vi "Auto_Path Tracking_edit.vi"() -> ()   [LabVIEW 2020]
uses:
  <vilib>/Utility/file.llb/Read Delimited Spreadsheet (DBL).vi
  <vilib>/Instr/_visa.llb/VISA Configure Serial Port (Instr).vi
panel:
  in  "Tab Control":enum32{"GPS", "LiDAR (TRUE)", "ETC"}(tab)
  out "XYGraph":cluster{"array":dbl[], "array":dbl[]}[](graph)
  in  "COM":refnum<visa-resource-name>
  out "도분초(lon)":string
  out "도(lon)":string
  out "도분초(lat)":string
  out "도(lat)":string
  out "Latitude":dbl
  out "Longtitude":dbl
  out "UTC":dbl
  out "TM_X":dbl format="%#_6f"
  out "TM_Y":dbl format="%#_6f"
  in  "Refresh 2":bool
  out "WP_no. 2":i32
  out "Satellited Used":string
  out "Fix Position":string
  out "True_Heading":dbl
  out "velocity":dbl
  out "read buffer":string
  out "Safe Box Plotting":cluster{dbl[], dbl[]}[](graph)
  out "Clustering graph":T1(graph)
  out "XY graph":cluster{"X":dbl, "Y":dbl}[](graph)
  out "Box Point Array":cluster{dbl[], dbl[]}[](array[cluster])
  out "XY DATA":cluster{"X":dbl, "Y":dbl}[](array[cluster])
  out "Path_Vel_arr 2":dbl[](array[numeric])
  out "Path_long_arr 2":dbl[](array[numeric])
  out "Path_lat_arr 2":dbl[](array[numeric])
  out "x_lat_path 2":dbl[](array[numeric])
  out "y_long_path 2":dbl[](array[numeric])
  out "vel. path 2":dbl[](array[numeric])
  in  "?":enum32{"State", "ETC"}(tab)
  in  "stop":bool
  in  "file path (dialog if empty)":path=path "C:/Users/Mondicht Shin/Desktop/ERP42_Auto_TEST/RDDF_3_수정.txt" caption="RDDF"
  out "XY Graph":T2(graph)
  in  "Refresh":bool
  in  "A/M":bool=TRUE
  in  "Serial Name":refnum<visa-resource-name>="COM8"
  out "ERP_Serial_DATA(RAW)":string
  in  "Vel":dbl=4.0 format="%#_13g"
  out "Index(near vehicle)":i32
  out "WP_no.":i32
  out "Tracking_Error(m)":dbl
  out "x_lat_path":dbl[](array[numeric])
  out "y_long_path":dbl[](array[numeric])
  out "vel. path":dbl[](array[numeric])
  out "Path_Vel_arr":dbl[](array[numeric])
  out "Path_long_arr":dbl[](array[numeric])
  out "Path_lat_arr":dbl[](array[numeric])
  out "ERP_Receive":T3
  out "Steer_CMD(Deg)":dbl
  out "CMD_2_ERP":T4
  out "Brake":u8
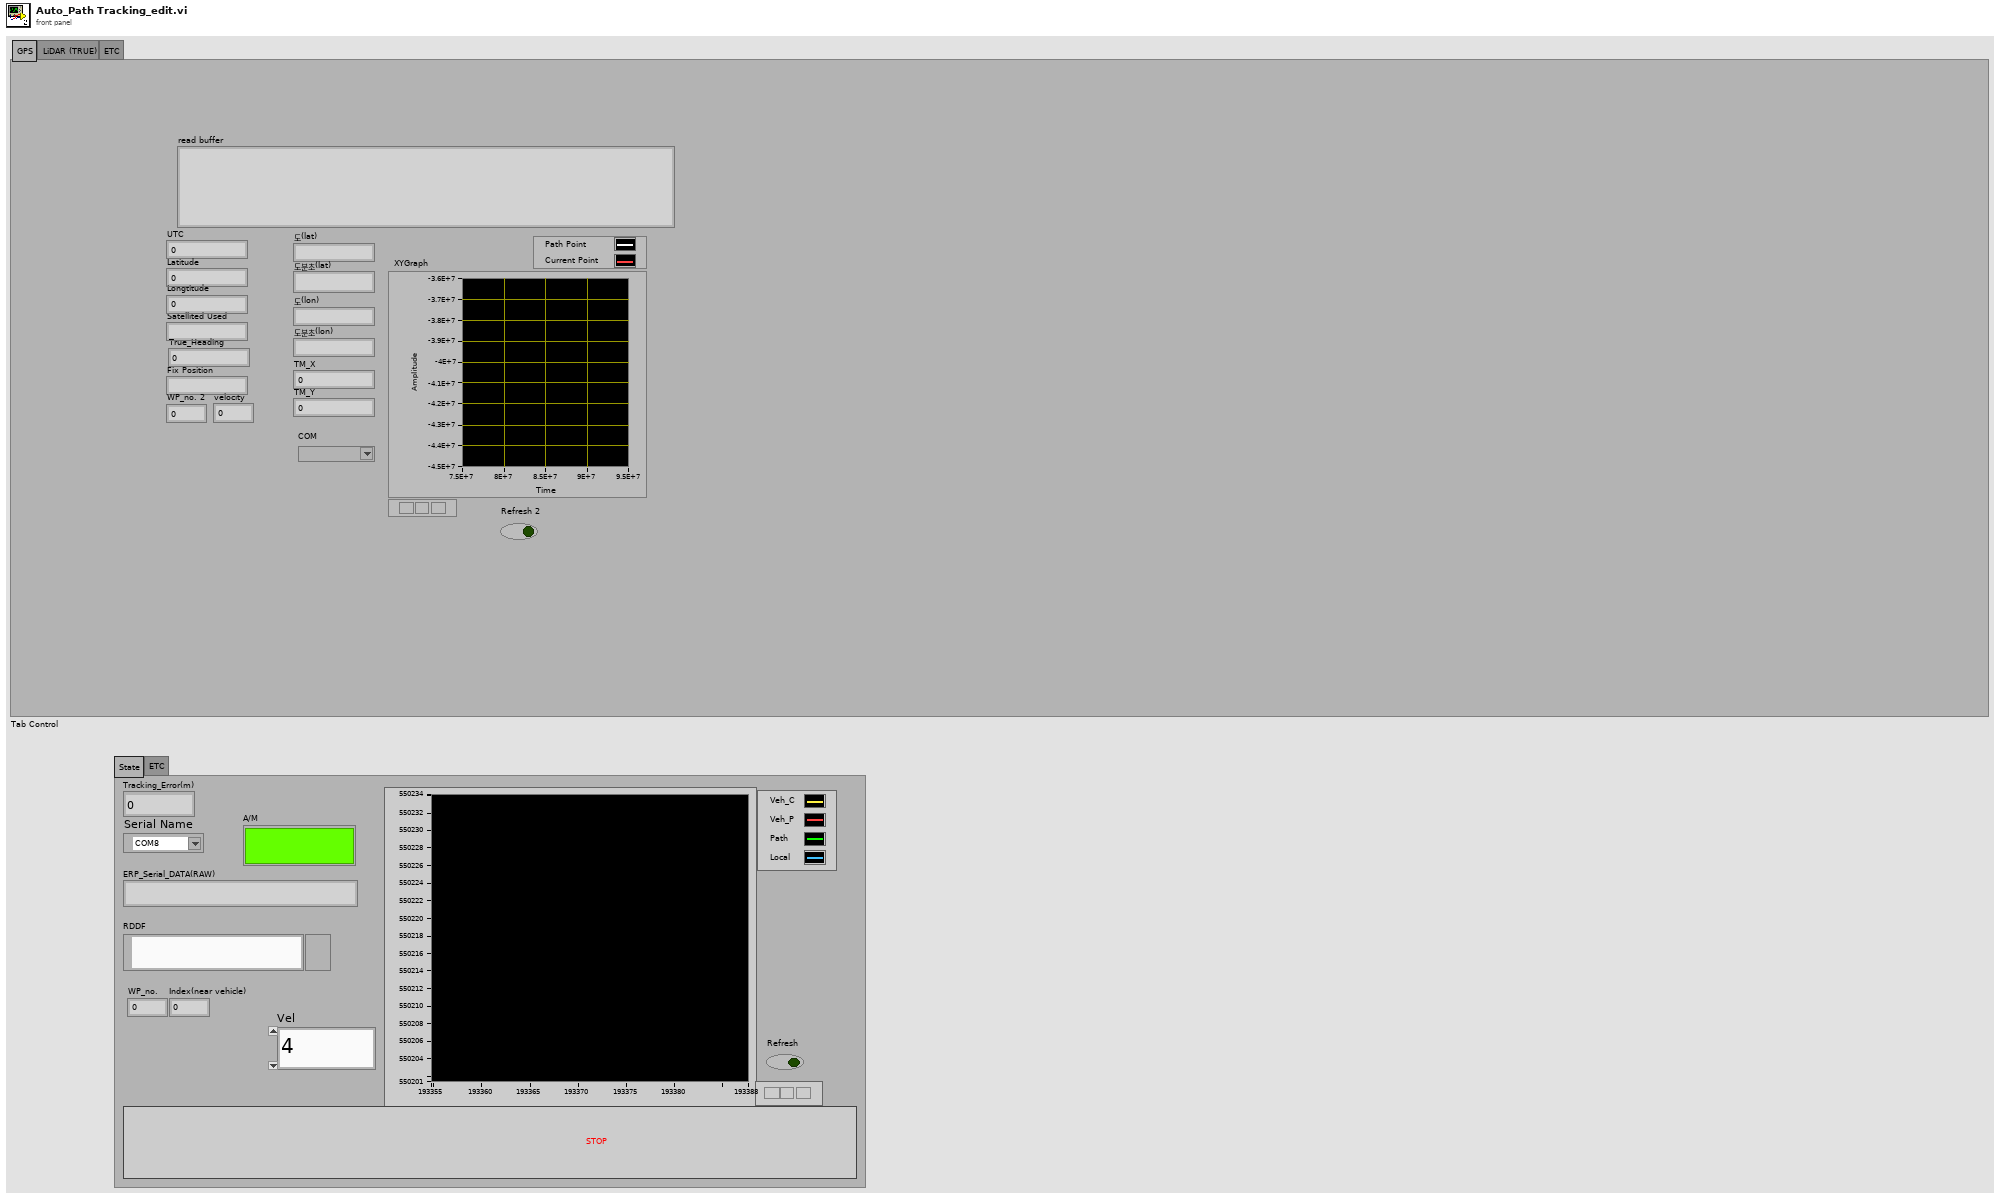
[diagram p1: front panel]
types:
  T1 = cluster{"최종 클러스터링 배열":cluster{"X":dbl, "Y":dbl}[]}[]
  T2 = cluster{"y_long_path":dbl[], "x_lat_path":dbl[]}[]
  T3 = cluster{"AorM":u8, "E-Stop":u8, "F_B":u8, "Speed":u16, "Steer":i16, "Brake":u8, "Encoder":u8, "Encoder 2":u8, "Encoder 3":u8, "Encoder 4":u8, "ALIVE":u8, "ETX_0":u8, "ETX_0 2":u8}
  T4 = cluster{"F/B":u8, "Speed":u16, "Steer":i16, "A/M":u8, "Brake":u8}
  T5 = cluster{"Path_long_arr":dbl[], "Path_lat_arr":dbl[]}
  T6 = cluster{"Path_long_arr":dbl[], "Path_lat_arr":dbl[]}[]
  T7 = cluster{"S":u8, "T":u8, "X":u8, "AorM":u8, "E-Stop":u8, "F_B":u8, "Speed":u16, "Steer":i16, "Brake":u8, "ALIVE":u8, "ETX_0":u8, "ETX_0 2":u8}
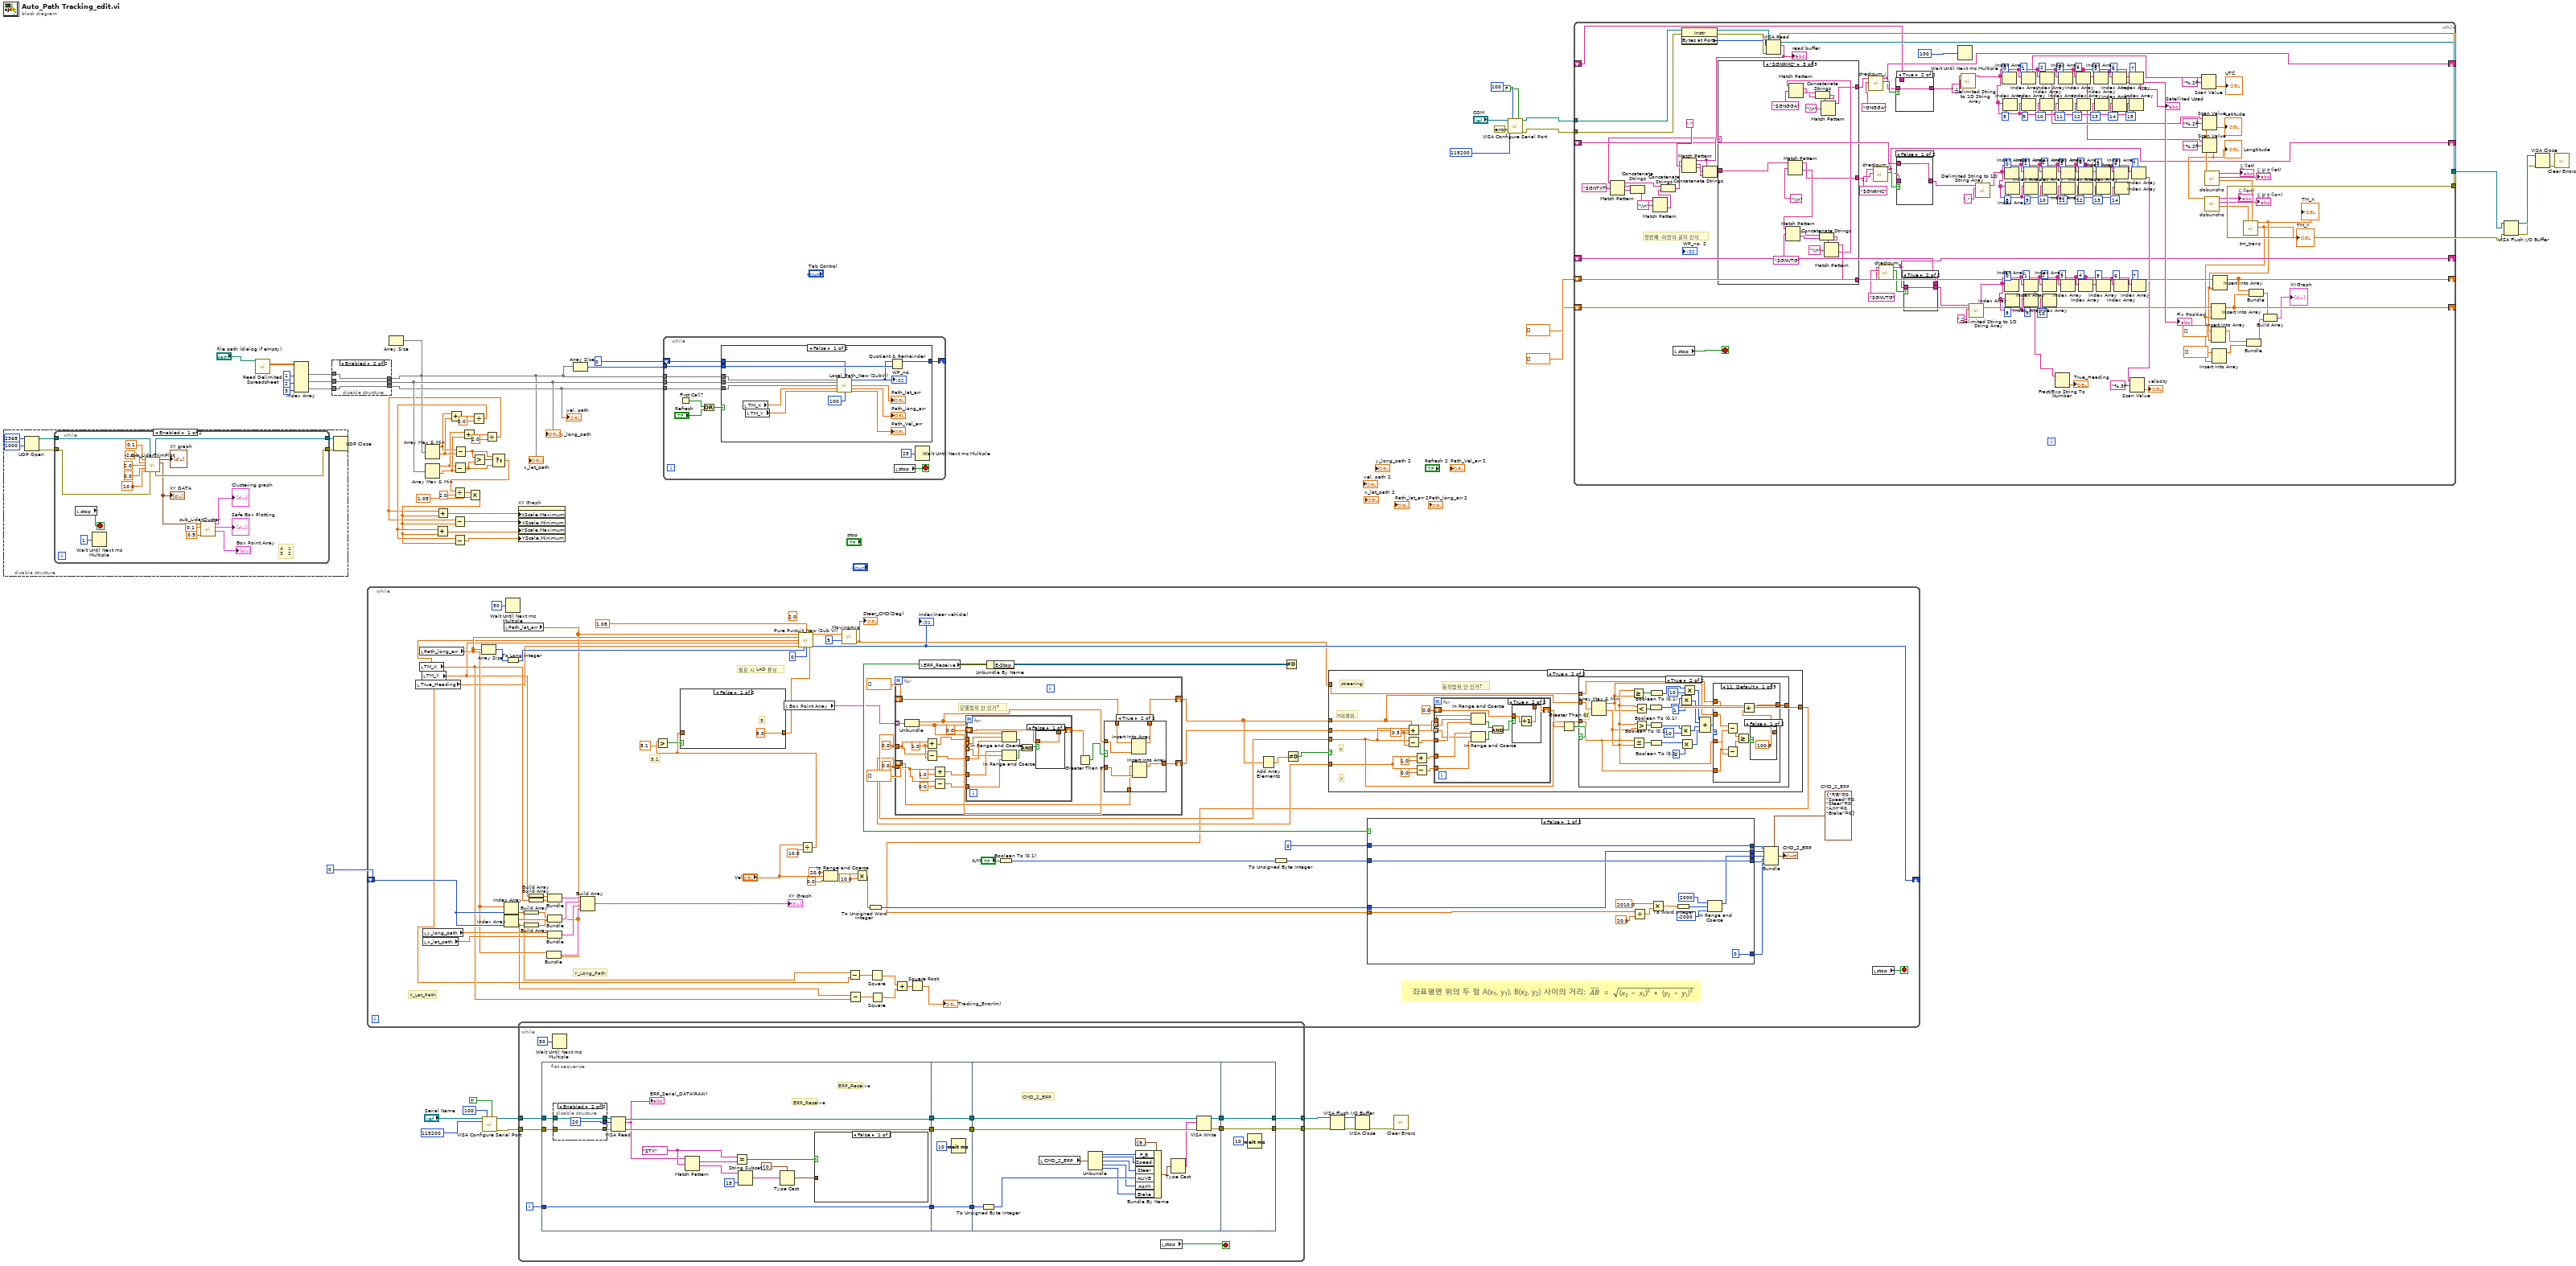
[diagram p0: block diagram]
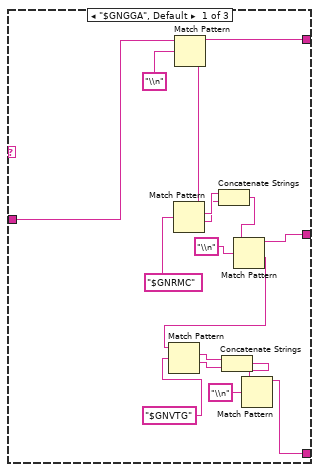
[diagram p5: hidden frame]
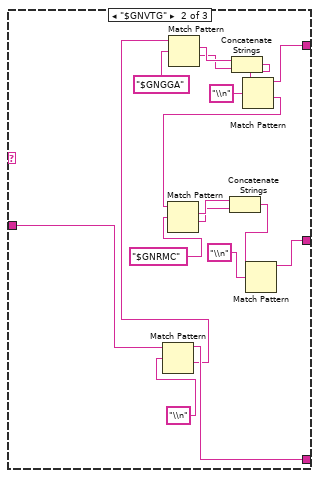
[diagram p6: hidden frame]
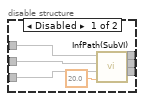
[diagram p8: hidden frame]
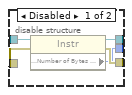
[diagram p9: hidden frame]
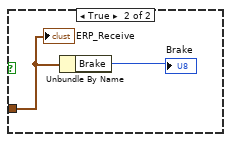
[diagram p10: hidden frame]
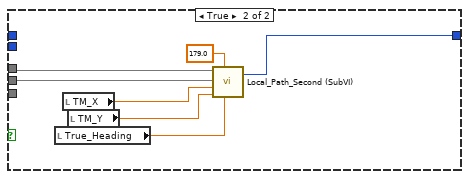
[diagram p11: hidden frame]
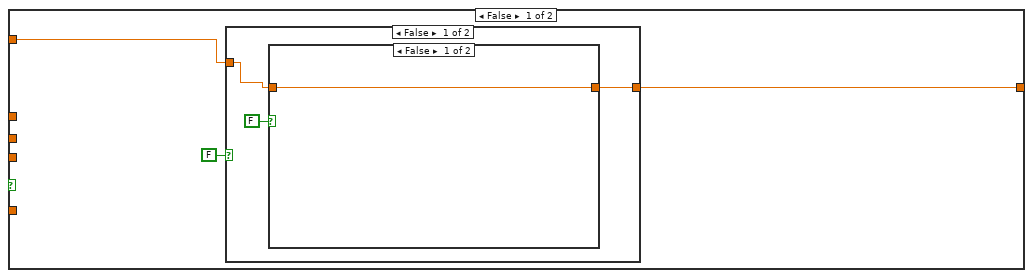
[diagram p12: hidden frame]
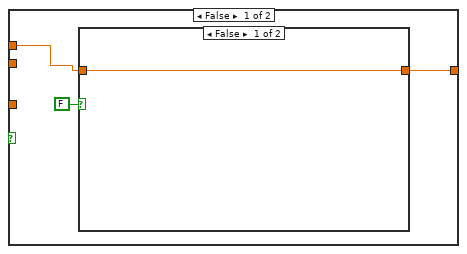
[diagram p16: hidden frame]
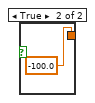
[diagram p18: hidden frame]
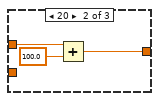
[diagram p19: hidden frame]
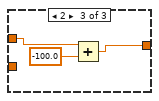
[diagram p20: hidden frame]
diagram:
  n1 = disable-structure shown="Enabled" {
    frame Enabled {
      n2 = UDP Open(9:1000 ("타임아웃 ms (25000)"), 11:u16 2368 ("포트")) -> (port=w64:refnum<k16>, 0:w65:errorcluster)  [unwired: 3 in, 1 out]
      n3 = while {
        tunnel: w64 -> [w79]
        tunnel: w65 -> [w78]
        tunnel: [w77] -> w63
        tunnel: [w76] -> w62
        stop <- w70 stop-if-true
        # "4   1\n3   2"
        n4 = local read "stop"() -> (w70:bool)
        n5 = Wait Until Next ms Multiple(millisecond multiple=u32 1 ("ms 배수")) -> ()  [unwired: 1 out]
        n6 = call "sub_LidarTrimPlot.vi"("R_min"=0.1, "UDP 네트워크 연결 입력"=w79, "x-"=-2.0, "x+"=2.0, "y-"=0.0, "y+"=10.0, "에러 입력(에러 없음)"=w78) -> ("UDP 네트워크 연결 출력"=w77:refnum<k16>, "Point Cloud Plotting"=→"XY graph":cluster{"X":dbl, "Y":dbl}[], "trim XY DATA"=w74:cluster{"X":dbl, "Y":dbl}[], "에러 출력"=w76:errorcluster)  [unwired: 5 in]
        "XY DATA" <- w74
        n7 = call "sub_LidarCluster.vi"("Box Offset"=0.5, "군집원소 간 거리(threshold)"=0.1, "XY DATA"=w74) -> ("Box Point Array"=→"Box Point Array":cluster{dbl[], dbl[]}[], "Safe Box Plotting"=→"Safe Box Plotting":cluster{dbl[], dbl[]}[], "Cluster Plotting"=→"Clustering graph":T1)  [unwired: 6 in]
      }
      n8 = UDP Close(connection ID=w63, 8:w62) -> ()  [unwired: 2 out]
    }
    frame Disabled {
    }
  }
  n9 = call-poly <vilib>:"Read Delimited Spreadsheet.vi"("file path (dialog if empty)"="file path (dialog if empty)") -> ("all rows"=w29:dbl[][])  [unwired: 9 in, 5 out]
  n10 = Index Array(array=w29, index (col) #1=1 ("비활성화된 인덱스 (열)"), index (col) #2=2 ("인덱스 (열)"), index (col) #3=3 ("인덱스 (열)")) -> (element #1=w58:dbl[], element #2=w57:dbl[], element #3=w56:dbl[])  [unwired: 3 in]
  n11 = disable-structure shown="Enabled" {
    disable-tunnel: w58 -> [w92 w95]
    disable-tunnel: w57 -> [w91 w94]
    disable-tunnel: w56 -> [w90 w93]
    disable-tunnel: [w89 w94] -> w33
    disable-tunnel: [w88 w93] -> w31
    disable-tunnel: [w87 w95] -> w30
    frame Disabled {
      n12 = call "InfPath(SubVI).vi"("Mod dist."=20.0, "vel."=w90, "y_long"=w91, "x_lat"=w92) -> ("vel. path"=w88:dbl[], "y_long_path"=w89:dbl[], "x_lat_path"=w87:dbl[])  [unwired: 1 out]
    }
    frame Enabled {
    }
  }
  "x_lat_path" <- w30
  "y_long_path" <- w33
  "vel. path" <- w31
  n13 = while {
    shift-right: [w153] -> _
    shift-left: 0 -> [w150]
    stop <- w159 stop-if-true
    w101 = 0.0 ("TM_Y")
    w102 = 0.0 ("TM_X")
    w125 = T4 {"F/B"=0, "Speed"=0, "Steer"=0, "A/M"=0, "Brake"=0}  # CMD_2_ERP
    (unwired) 2.0 ("L")
    # "5.1"
    # "X_Lat_Path"
    # "Y_Long_Path"
    # "필요 시 LAD 튜닝"
    n14 = local read "True_Heading"() -> (w146:dbl)
    n15 = local read "Path_long_arr"() -> (w122:dbl[])
    n16 = local read "TM_X"() -> (w107:dbl)
    n17 = local read "TM_Y"() -> (w106:dbl)
    n18 = local read "y_long_path"() -> (w130:dbl[])
    n19 = local read "x_lat_path"() -> (w129:dbl[])
    n20 = Array Size(array=w122) -> (size(s)=w154:i32)
    n21 = local read "Path_lat_arr"() -> (w121:dbl[])
    n22 = Index Array(array=w122, index=w150) -> (element=w112:dbl)
    n23 = Index Array(array=w121, index=w150) -> (element=w111:dbl)
    n24 = Wait Until Next ms Multiple(millisecond multiple=u32 50 ("ms 배수")) -> ()  [unwired: 1 out]
    n25 = To Long Integer(number=w154) -> (32bit integer=w152:i32)
    n26 = Build Array(w112) -> (w161:dbl[])
    n27 = Build Array(w111) -> (w160:dbl[])
    n28 = Build Array(w106) -> (w163:dbl[])
    n29 = Build Array(w107) -> (w162:dbl[])
    n30 = Bundle("Path_long_arr"=w122, "Path_lat_arr"=w121) -> (w142:T5)  [unwired: 1 in]
    n31 = Bundle(w163, w162) -> (w148:cluster{dbl[], dbl[]})  [unwired: 1 in]
    n32 = Bundle(w161, w160) -> (w147:cluster{dbl[], dbl[]})  [unwired: 1 in]
    n33 = Bundle("y_long_path"=w130, "x_lat_path"=w129) -> (w149:cluster{"y_long_path":dbl[], "x_lat_path":dbl[]})  [unwired: 1 in]
    n34 = Build Array(w148, w147, w149, w142) -> (→"XY Graph":T6)
    n35 = local read "Box Point Array"() -> (w108:cluster{dbl[], dbl[]}[])
    n36 = Divide(x="Vel", y=10.0) -> (x/y=w143:dbl)
    n37 = Greater?(x=w143, y=5.1) -> (0:w110:bool)
    n38 = case shown="False" w110 {
      tunnel: w143 -> [_ w294]
      tunnel: [5.0 w293] -> w145
      frame False {
        # "5"
      }
      frame True {
        w295 = 3.7978021978021976  # intercept
        w297 = 0.23736263736263735  # slope
        n39 = Multiply(x=w297, y=w294) -> (x*y=w296:dbl)
        n40 = Add(x=w296, y=w295) -> (x+y=w293:dbl)
      }
    }
    n41 = call "Pure Pursuit_New (Sub VI).vi"("x_lat_path"=w121, "L"=1.08, "y_long_path"=w122, "X_Current"=w107, "Y_Current"=w106, "Heading_Current"=w146, "#pnt"=w152, "WP no_pre"=0, "LAD"=w145) -> ("Steer_CMD(Deg)"=w120:dbl, "Index(near vehicle)"=w153:i32)  [unwired: 5 in]
    "Index(near vehicle)" <- w153
    n42 = In Range and Coerce(upper limit=20.0 ("상위 리미트"), x="Vel", lower limit=0.0 ("하위 리미트")) -> (coerced(x)=w134:dbl)  [unwired: 1 out]
    n43 = call "MovingAvg.vi"("입력"=w120, "이동평균을 구할 자료의 개수"=u16 5) -> ("이동평균"=w100:dbl)  [unwired: 2 out]
    "Steer_CMD(Deg)" <- w100
    n44 = Subtract(x=w112, y=w106) -> (x-y=w117:dbl)
    n45 = Subtract(x=w111, y=w107) -> (x-y=w116:dbl)
    n46 = Multiply(x=w134, y=10.0) -> (x*y=w132:dbl)
    n47 = To Unsigned Word Integer(number=w132) -> (unsigned 16bit integer=w138:u16)
    n48 = Square(x=w117) -> (x^2=w115:dbl)
    n49 = Square(x=w116) -> (x^2=w114:dbl)
    n50 = for {
      tunnel: w108 -> [w269] mode=indexing
      tunnel: w102 -> [w262]
      tunnel: w101 -> [w260]
      shift-right: [w254] -> w98
      shift-left: dbl[] [] -> [w255]
      shift-right: [w252] -> w103
      shift-left: dbl[] [] -> [w251]
      w261 = 1.0 ("y")
      # "모델범위 안 인가?"
      n51 = Unbundle(w269) -> (w256:dbl[], w253:dbl[])
      n52 = Add(x=w262, y=w261) -> (x+y=w266:dbl)
      n53 = Subtract(x=w262, y=w261) -> (x-y=w265:dbl)
      n54 = Add(x=w260, y=1.0) -> (x+y=w264:dbl)
      n55 = Subtract(x=w260, y=0.0) -> (x-y=w263:dbl)
      n56 = for {
        tunnel: w256 -> [w286] mode=indexing
        tunnel: w253 -> [w283] mode=indexing
        tunnel: w266 -> [w288]
        tunnel: w265 -> [w287]
        tunnel: w264 -> [w285]
        tunnel: w263 -> [w284]
        shift-right: [w278] -> w259
        shift-left: 0.0 -> [w279]
        n57 = In Range and Coerce(upper limit=w288, x=w286, lower limit=w287) -> (In Range?=w282:bool)  [unwired: 1 out]
        n58 = In Range and Coerce(upper limit=w285, x=w283, lower limit=w284) -> (In Range?=w281:bool)  [unwired: 1 out]
        n59 = And(x=w282, y=w281) -> (x .and. y?=w280:bool)
        n60 = case shown="False" w280 {
          tunnel: w279 -> [w289 w291]
          tunnel: [w289 w290] -> w278
          frame False {
          }
          frame True {
            n61 = Increment(x=w291) -> (x+1=w290:dbl)
          }
        }
      }
      n62 = Greater Than 0?(x=w259) -> (x > 0?=w257:bool)
      n63 = case shown="True" w257 {
        tunnel: w256 -> [_ w277]
        tunnel: w255 -> [w271 w276]
        tunnel: [w271 w275] -> w254
        tunnel: w253 -> [_ w274]
        tunnel: [w270 w273] -> w252
        tunnel: w251 -> [w270 w272]
        frame False {
        }
        frame True {
          n64 = Insert Into Array(array=w276, new element=w277) -> (w275:dbl[])  [unwired: 1 in]
          n65 = Insert Into Array(array=w272, new element=w274) -> (w273:dbl[])  [unwired: 1 in]
        }
      }
    }
    n66 = Add(x=w115, y=w114) -> (x+y=w113:dbl)
    n67 = Square Root(x=w113) -> (sqrt(x)=→"Tracking_Error(m)":dbl)
    n68 = local read "ERP_Receive"() -> (w156:T3)
    n69 = Unbundle By Name(w156) -> ("E-Stop"=w157:u8)
    n70 = Boolean To (0,1)(Boolean="A/M") -> (0, 1=w141:i16)
    n71 = Add Array Elements(numeric array=w98) -> (sum=w97:dbl)
    n72 = To Unsigned Byte Integer(number=w141) -> (unsigned 8bit integer=w123:u8)
    n73 = Not Equal To 0?(x=w157) -> (x != 0?=w137:bool)
    n74 = Not Equal To 0?(x=w97) -> (x != 0?=w96:bool)
    n75 = case shown="True" w96 {
      tunnel: w100 -> [w169 w191]
      tunnel: [w168 w190] -> w99
      tunnel: w98 -> [_ w176]
      tunnel: w103 -> [_ w189]
      tunnel: w102 -> [_ w177]
      tunnel: w101 -> [_ w185]
      frame False {
        n76 = case shown="False" FALSE {
          tunnel: w169 -> [w172 w175]
          tunnel: [w171 w175] -> w168
          frame False {
            n77 = case shown="False" FALSE {
              tunnel: w172 -> [w173 w174]
              tunnel: [w173 w174] -> w171
              frame False {
              }
              frame True {
              }
            }
          }
          frame True {
          }
        }
      }
      frame True {
        w186 = 0.3 ("y")
        # "y"
        # "x"
        # "streering"
        # "x어레이"
        # "동작범위 안 인가?"
        n78 = Add(x=w177, y=w186) -> (x+y=w184:dbl)
        n79 = Subtract(x=w177, y=w186) -> (x-y=w183:dbl)
        n80 = Add(x=w185, y=1.0) -> (x+y=w182:dbl)
        n81 = Subtract(x=w185, y=0.0) -> (x-y=w181:dbl)
        n82 = for {
          tunnel: w176 -> [w200] mode=indexing
          tunnel: w189 -> [w197] mode=indexing
          tunnel: w184 -> [w202]
          tunnel: w183 -> [w201]
          tunnel: w182 -> [w199]
          tunnel: w181 -> [w198]
          shift-right: [w194] -> w179
          shift-left: 0.0 -> [w193]
          n83 = In Range and Coerce(upper limit=w202, x=w200, lower limit=w201) -> (In Range?=w196:bool)  [unwired: 1 out]
          n84 = In Range and Coerce(upper limit=w199, x=w197, lower limit=w198) -> (In Range?=w195:bool)  [unwired: 1 out]
          n85 = And(x=w196, y=w195) -> (x .and. y?=w192:bool)
          n86 = case shown="True" w192 {
            tunnel: w193 -> [w203 w205]
            tunnel: [w203 w204] -> w194
            frame False {
            }
            frame True {
              n87 = Increment(x=w205) -> (x+1=w204:dbl)
            }
          }
        }
        n88 = Greater Than 0?(x=w179) -> (x > 0?=w178:bool)
        n89 = case shown="True" w178 {
          tunnel: w191 -> [w208 w216]
          tunnel: [w207 w215] -> w190
          tunnel: w177 -> [_ w214]
          tunnel: w176 -> [_ w213]
          frame False {
            n90 = case shown="False" FALSE {
              tunnel: w208 -> [w209 w210]
              tunnel: [w209 w210] -> w207
              frame False {
              }
              frame True {
              }
            }
          }
          frame True {
            # "x"
            n91 = Array Max & Min(array=w213) -> (max value=w212:dbl, min value=w211:dbl)  [unwired: 2 out]
            n92 = Greater Or Equal?(x=w214, y=w212) -> (x >= y?=w233:bool)
            n93 = Less Or Equal?(x=w214, y=w211) -> (x <= y?=w232:bool)
            n94 = Less?(x=w214, y=w212) -> (x < y?=w218:bool)
            n95 = Greater?(x=w214, y=w211) -> (0:w217:bool)
            n96 = Boolean To (0,1)(Boolean=w218) -> (0, 1=w225:i16)
            n97 = Boolean To (0,1)(Boolean=w217) -> (0, 1=w227:i16)
            n98 = Boolean To (0,1)(Boolean=w232) -> (0, 1=w226:i16)
            n99 = Boolean To (0,1)(Boolean=w233) -> (0, 1=w224:i16)
            n100 = Multiply(x=w227, y=i16 10) -> (x*y=w221:i16)
            n101 = Multiply(x=w225, y=i16 1) -> (x*y=w222:i16)
            n102 = Multiply(x=w226, y=i16 1) -> (x*y=w220:i16)
            n103 = Multiply(x=w224, y=i16 10) -> (x*y=w223:i16)
            n104 = Compound Arithmetic op=ADD(w223, w222, w221, w220) -> (w219:i16)
            n105 = case shown="11, Default" w219 {
              tunnel: w216 -> [w236 w247 w248]
              tunnel: [w234 w245 w249] -> w215
              tunnel: w212 -> [w241 _ _]
              tunnel: w211 -> [w240 _ _]
              tunnel: w214 -> [w242 _ _]
              frame 11, Default {
                n106 = Subtract(x=w241, y=w242) -> (x-y=w239:dbl)
                n107 = Subtract(x=w242, y=w240) -> (x-y=w238:dbl)
                n108 = Greater Or Equal?(x=w239, y=w238) -> (x >= y?=w237:bool)
                n109 = case shown="False" w237 {
                  tunnel: [100.0 -100.0] -> w235
                  frame False {
                  }
                  frame True {
                  }
                }
                n110 = Add(x=w236, y=w235) -> (x+y=w234:dbl)
              }
              frame 20 {
                n111 = Add(x=w247, y=100.0) -> (x+y=w245:dbl)
              }
              frame 2 {
                n112 = Add(x=w248, y=-100.0) -> (x+y=w249:dbl)
              }
            }
          }
        }
      }
    }
    n113 = case shown="False" w137 {
      tunnel: u8 0 -> [w310 _]
      tunnel: [w310 w312] -> w166
      tunnel: [w307 w312] -> w165
      tunnel: [w299 w312] -> w164
      tunnel: [w309 w312] -> w140
      tunnel: w123 -> [w309 _]
      tunnel: w99 -> [w308 _]
      tunnel: w138 -> [w307 _]
      tunnel: [u8 0 u8 200] -> w126
      frame False {
        n114 = Divide(x=w308, y=20.0) -> (x/y=w305:dbl)
        n115 = Multiply(x=2010.0, y=w305) -> (x*y=w304:dbl)
        n116 = To Word Integer(number=w304) -> (16bit integer=w306:i16)
        n117 = In Range and Coerce(upper limit=i16 2000 ("상위 리미트"), x=w306, lower limit=i16 -2000 ("하위 리미트")) -> (coerced(x)=w299:i16)  [unwired: 1 out]
      }
      frame True {
        w312 = u8 0
      }
    }
    n118 = Bundle(cluster=w125, "F/B"=w166, "Speed"=w165, "Steer"=w164, "A/M"=w140, "Brake"=w126) -> (→"CMD_2_ERP":T4)
    n119 = local read "stop"() -> (w159:bool)
  }
  n120 = Array Size(array=w30) -> ()  [unwired: 1 out]
  n121 = Array Max & Min(array=w33) -> (max value=w44:dbl, min value=w43:dbl)  [unwired: 2 out]
  n122 = Array Max & Min(array=w30) -> (max value=w50:dbl, min value=w49:dbl)  [unwired: 2 out]
  n123 = Add(x=w50, y=w49) -> (x+y=w47:dbl)
  n124 = Subtract(x=w44, y=w43) -> (x-y=w53:dbl)
  n125 = Subtract(x=w50, y=w49) -> (x-y=w54:dbl)
  n126 = Add(x=w44, y=w43) -> (x+y=w46:dbl)
  n127 = Divide(x=w47, y=2.0) -> (x/y=w40:dbl)
  n128 = Greater?(x=w54, y=w53) -> (0:w55:bool)
  n129 = call-poly "VISA Configure Serial Port"("VISA resource name"="Serial Name", "timeout (10sec)"=u32 100, "Enable Termination\nChar (T)"=TRUE ("Enable Termination\nChar (T)"), "baud rate (9600)"=u32 115200) -> ("VISA resource name out"=w17:refnum<visa-resource-name>, "error out"=w16:errorcluster)  [unwired: 10 in]
  n130 = Divide(x=w46, y=2.0) -> (x/y=w27:dbl)
  n131 = Select(t=w54, s=w55, f=w53) -> (s? t:f=w51:dbl)
  n132 = Divide(x=w51, y=2.0) -> (x/y=w42:dbl)
  n133 = Multiply(x=w42, y=1.05) -> (x*y=w39:dbl)
  n134 = Add(x=w40, y=w39) -> (x+y=w37:dbl)
  n135 = Add(x=w27, y=w39) -> (x+y=w35:dbl)
  n136 = Subtract(x=w27, y=w39) -> (x-y=w36:dbl)
  n137 = Subtract(x=w40, y=w39) -> (x-y=w38:dbl)
  n138 = property on="XY Graph" class="XYGraph (strict)"("XScale.Maximum"=w35, "XScale.Minimum"=w36, "YScale.Maximum"=w37, "YScale.Minimum"=w38) -> ()  [unwired: 2 in, 2 out]
  n139 = while {
    tunnel: w17 -> [w326]
    tunnel: w16 -> [w325]
    tunnel: [w323] -> w19
    tunnel: [w322] -> w18
    i -> [w324]
    stop <- w315 stop-if-true
    n140 = flat-sequence {
      tunnel: w326 -> [w344]
      tunnel: w325 -> [w343]
      tunnel: [w342] -> w321
      tunnel: [w341] -> w319
      tunnel: w324 -> [w340]
      tunnel: [w340] -> w317
      tunnel: w321 -> [w358]
      tunnel: [w358] -> w320
      tunnel: w319 -> [w357]
      tunnel: [w357] -> w318
      tunnel: w317 -> [w356]
      tunnel: [w356] -> w316
      tunnel: w320 -> [w371]
      tunnel: w318 -> [w370]
      tunnel: w316 -> [w368]
      tunnel: [w367] -> w314
      tunnel: [w366] -> w313
      tunnel: [w375] -> w322
      tunnel: [w376] -> w323
      tunnel: w314 -> [w376]
      tunnel: w313 -> [w375]
      frame #0 {
        w334 = "STX" ("검색 문자열/문자 (-)")
        # "ERP_Receive"
        # "ERP_Receive"
        n141 = disable-structure shown="Enabled" {
          disable-tunnel: w344 -> [w349 w351]
          disable-tunnel: w343 -> [w348 w352]
          disable-tunnel: [w347 w352] -> w339
          disable-tunnel: [w346 u32 20 ("timeout (10sec)")] -> w338
          disable-tunnel: [w345 w351] -> w337
          frame Disabled {
            n142 = property class="Instr"(reference=w349, error in=w348) -> (reference out=w345:refnum<visa-resource-name>, error out=w347:errorcluster, "Serial Settings:Number of Bytes at Serial Port"=w346:u32)
          }
          frame Enabled {
          }
        }
        n143 = VISA Read(VISA resource name=w337, byte count=w338, error in (no error)=w339) -> (VISA resource name out=w342:refnum<visa-resource-name>, read buffer=w332:string, error out=w341:errorcluster)  [unwired: 1 out]
        "ERP_Serial_DATA(RAW)" <- w332
        n144 = Match Pattern(string=w332, regular expression=w334) -> (match substring=w333:string, after substring=w336:string)  [unwired: 1 in, 2 out]
        n145 = Equal?(x=w334, y=w333) -> (x = y?=w331:bool)
        n146 = String Subset(string=w336, length (rest)=15 ("길이(나머지)")) -> (substring=w330:string)  [unwired: 1 in]
        n147 = Type Cast(type=T3 {"AorM"=0, "E-Stop"=0, "F_B"=0, "Speed"=0, "Steer"=0, "Brake"=0, "Encoder"=0, "Encoder 2"=0, "Encoder 3"=0, "Encoder 4"=0, "ALIVE"=0, "ETX_0"=13, "ETX_0 2"=10}, x=w330) -> (*(type *) &x=w329:T3)
        n148 = case shown="False" w331 {
          tunnel: w329 -> [_ w354]
          frame False {
          }
          frame True {
            n149 = Unbundle By Name(w354) -> ("Brake"=→"Brake":u8)
            "ERP_Receive" <- w354
          }
        }
      }
      frame #1 {
        n150 = Wait (ms)(milliseconds to wait=u32 10 ("대기 시간(ms)")) -> ()  [unwired: 1 out]
      }
      frame #2 {
        # "CMD_2_ERP"
        n151 = To Unsigned Byte Integer(number=w368) -> (unsigned 8bit integer=w373:u8)
        n152 = local read "CMD_2_ERP"() -> (w360:T4)
        n153 = Unbundle(w360) -> ("F/B"=w365:u8, "Speed"=w364:u16, "Steer"=w363:i16, "A/M"=w361:u8, "Brake"=w359:u8)
        n154 = Bundle By Name(cluster=T7 {"S"=83, "T"=84, "X"=88, "AorM"=0, "E-Stop"=0, "F_B"=0, "Speed"=0, "Steer"=0, "Brake"=0, "ALIVE"=0, "ETX_0"=13, "ETX_0 2"=10}, "F_B"=w365, "Speed"=w364, "Steer"=w363, "ALIVE"=w373, "AorM"=w361, "Brake"=w359) -> (w372:T7)
        n155 = Type Cast(x=w372) -> (*(type *) &x=w369:string)  [unwired: 1 in]
        n156 = VISA Write(VISA resource name=w371, write buffer=w369, error in (no error)=w370) -> (VISA resource name out=w367:refnum<visa-resource-name>, error out=w366:errorcluster)  [unwired: 1 out]
      }
      frame #3 {
        n157 = Wait (ms)(milliseconds to wait=u32 10 ("대기 시간(ms)")) -> ()  [unwired: 1 out]
      }
    }
    n158 = Wait Until Next ms Multiple(millisecond multiple=u32 50 ("ms 배수")) -> ()  [unwired: 1 out]
    n159 = local read "stop"() -> (w315:bool)
  }
  n160 = Array Size(array=w30) -> (size(s)=w32:i32)
  n161 = while {
    tunnel: w30 -> [w386]
    tunnel: w33 -> [w385]
    tunnel: w31 -> [w383]
    tunnel: w32 -> [w382]
    shift-right: [w381] -> _
    shift-left: 0 ("Index0") -> [w384]
    stop <- w387 stop-if-true
    n162 = First Call?() -> (First Call?: T/F=w379:bool)
    n163 = Or(x=w379, y="Refresh") -> (x .or. y?=w380:bool)
    n164 = case shown="False" w380 {
      tunnel: w386 -> [w388 w407]
      tunnel: w385 -> [w390 w406]
      tunnel: w384 -> [w395 _]
      tunnel: w383 -> [w389 _]
      tunnel: w382 -> [w399 _]
      tunnel: [w400 w401] -> w381
      frame False {
        n165 = local read "TM_X"() -> (w398:dbl)
        n166 = local read "TM_Y"() -> (w397:dbl)
        n167 = call "Local_Path_New (SubVI).vi"("x_lat_arr"=w388, "WP no_pre"=w395, "y_long_arr"=w390, "vel_arr"=w389, "x_lat_c"=w398, "y_long_c"=w397, "# of pnt"=100) -> ("INDEX(Near Point)"=w391:i32, "Lat(Local)"=→"Path_lat_arr":dbl[], "Long(Local)"=→"Path_long_arr":dbl[], "Vel(Local)"=→"Path_Vel_arr":dbl[])  [unwired: 5 in]
        "WP_no." <- w391
        n168 = Quotient & Remainder(x=w391, y=w399) -> (x-y*floor(x/y)=w400:i32)  [unwired: 1 out]
      }
      frame True {
        n169 = local read "True_Heading"() -> (w403:dbl)
        n170 = local read "TM_X"() -> (w405:dbl)
        n171 = local read "TM_Y"() -> (w404:dbl)
        n172 = call "Local_Path_Second (SubVI).vi"("heading_deg"=w403, "heading_limit"=179.0, "y_long"=w404, "x_lat"=w405, "Y_long_path"=w406, "X_lat_path"=w407) -> ("Index(near vehicle)"=w401:i32)  [unwired: 1 out]
      }
    }
    n173 = local read "stop"() -> (w387:bool)
    n174 = Wait Until Next ms Multiple(millisecond multiple=u32 25) -> ()  [unwired: 1 out]
  }
  n175 = VISA Flush I/O Buffer(VISA resource name=w19, error in (no error)=w18) -> (VISA resource name out=w20:refnum<visa-resource-name>, error out=w21:errorcluster)  [unwired: 1 in]
  n176 = VISA Close(VISA resource name=w20, error in (no error)=w21) -> (error out=w15:errorcluster)
  n177 = call <vilib>:"Clear Errors.vi"("error in (no error)"=w15) -> ()  [unwired: 5 in, 2 out]
  n178 = call-poly "VISA Configure Serial Port"("VISA resource name"="COM", "timeout (10sec)"=u32 100, "Enable Termination\nChar (T)"=FALSE ("Enable Termination\nChar (T)"), "baud rate (9600)"=u32 115200 ("baud rate (115200)"), "error in (no error)"=errorcluster {"status"=FALSE, "code"=0, "source"=""}) -> ("VISA resource name out"=w7:refnum<visa-resource-name>, "error out"=w6:errorcluster)  [unwired: 9 in]
  n179 = while {
    tunnel: w7 -> [w482]
    tunnel: w6 -> [w481]
    tunnel: [w471] -> w2
    tunnel: [w470] -> w1
    shift-right: [w433] -> _
    shift-left: _ -> [w453]
    shift-right: [w429] -> _
    shift-left: _ -> [w451]
    shift-right: [w426] -> _
    shift-left: _ -> [w449]
    shift-right: [w447] -> _
    shift-left: dbl[] [] -> [w448]
    shift-right: [w445] -> _
    shift-left: dbl[] [] -> [w446]
    stop <- w408 stop-if-true
    # "첫번째 ,이전의 글자 인식"
    n180 = local read "stop"() -> (w408:bool)
    n181 = property class="Instr"(reference=w482, error in=w481) -> (reference out=w480:refnum<visa-resource-name>, error out=w479:errorcluster, "Bytes at Port"=w469:u32)
    n182 = VISA Read(VISA resource name=w480, byte count=w469, error in (no error)=w479) -> (VISA resource name out=w471:refnum<visa-resource-name>, read buffer=w409:string, error out=w470:errorcluster)  [unwired: 1 out]
    "read buffer" <- w409
    n183 = Match Pattern(string=w409, regular expression="$GNTXT") -> (before substring=w412:string, match substring=w416:string, after substring=w415:string)  [unwired: 1 in, 1 out]
    n184 = Concatenate Strings(w416, w415) -> (w414:string)
    n185 = Match Pattern(string=w414, regular expression="\\n") -> (after substring=w411:string)  [unwired: 1 in, 3 out]
    n186 = Concatenate Strings(w412, w411) -> (w410:string)
    n187 = Match Pattern(string=w410, regular expression=",") -> (before substring=w463:string, match substring=w462:string, after substring=w461:string)  [unwired: 1 in, 1 out]
    n188 = Concatenate Strings(w463, w462, w461) -> (w464:string)
    n189 = case shown="\"$GNRMC\"" w463 {
      tunnel: w464 -> [w553 w570 w585]
      tunnel: [w545 w555 w584] -> w431
      tunnel: [w538 w568 w578] -> w427
      tunnel: [w552 w562 w572] -> w418
      frame "$GNGGA", Default {
        n190 = Match Pattern(string=w553, regular expression="\\n") -> (before substring=w552:string, after substring=w551:string)  [unwired: 1 in, 2 out]
        n191 = Match Pattern(string=w551, regular expression="$GNRMC") -> (match substring=w548:string, after substring=w547:string)  [unwired: 1 in, 2 out]
        n192 = Concatenate Strings(w548, w547) -> (w546:string)
        n193 = Match Pattern(string=w546, regular expression="\\n") -> (before substring=w545:string, after substring=w542:string)  [unwired: 1 in, 2 out]
        n194 = Match Pattern(string=w542, regular expression="$GNVTG") -> (match substring=w540:string, after substring=w539:string)  [unwired: 1 in, 2 out]
        n195 = Concatenate Strings(w540, w539) -> (w543:string)
        n196 = Match Pattern(string=w543, regular expression="\\n") -> (before substring=w538:string)  [unwired: 1 in, 3 out]
      }
      frame "$GNVTG" {
        n197 = Match Pattern(string=w570, regular expression="\\n") -> (before substring=w568:string, after substring=w567:string)  [unwired: 1 in, 2 out]
        n198 = Match Pattern(string=w567, regular expression="$GNGGA") -> (match substring=w564:string, after substring=w563:string)  [unwired: 1 in, 2 out]
        n199 = Concatenate Strings(w564, w563) -> (w565:string)
        n200 = Match Pattern(string=w565, regular expression="\\n") -> (before substring=w562:string, after substring=w561:string)  [unwired: 1 in, 2 out]
        n201 = Match Pattern(string=w561, regular expression="$GNRMC") -> (match substring=w557:string, after substring=w556:string)  [unwired: 1 in, 2 out]
        n202 = Concatenate Strings(w557, w556) -> (w558:string)
        n203 = Match Pattern(string=w558, regular expression="\\n") -> (before substring=w555:string)  [unwired: 1 in, 3 out]
      }
      frame "$GNRMC" {
        n204 = Match Pattern(string=w585, regular expression="\\n") -> (before substring=w584:string, after substring=w583:string)  [unwired: 1 in, 2 out]
        n205 = Match Pattern(string=w583, regular expression="$GNVTG") -> (match substring=w579:string, after substring=w580:string)  [unwired: 1 in, 2 out]
        n206 = Concatenate Strings(w579, w580) -> (w581:string)
        n207 = Match Pattern(string=w581, regular expression="\\n") -> (before substring=w578:string, after substring=w577:string)  [unwired: 1 in, 2 out]
        n208 = Match Pattern(string=w577, regular expression="$GNGGA") -> (match substring=w574:string, after substring=w573:string)  [unwired: 1 in, 2 out]
        n209 = Concatenate Strings(w574, w573) -> (w575:string)
        n210 = Match Pattern(string=w575, regular expression="\\n") -> (before substring=w572:string)  [unwired: 1 in, 3 out]
      }
    }
    n211 = call "checksum_i.vi"("check dataName"="GNGGA", "string"=w418) -> ("Boolean"=w434:bool, "String"=w433:string)  [unwired: 8 in]
    n212 = call "checksum_i.vi"("check dataName"="$GNRMC", "string"=w431) -> ("Boolean"=w430:bool, "String"=w429:string)  [unwired: 8 in]
    n213 = call "checksum_i.vi"("check dataName"="$GNVTG", "string"=w427) -> ("Boolean"=w425:bool, "String"=w426:string)  [unwired: 8 in]
    n214 = case shown="True" w434 {
      tunnel: [w536 w537] -> w454
      tunnel: w433 -> [_ w537]
      tunnel: w453 -> [w536 _]
      frame False {
      }
      frame True {
      }
    }
    n215 = case shown="False" w430 {
      tunnel: w429 -> [_ w535]
      tunnel: [w534 w535] -> w452
      tunnel: w451 -> [w534 _]
      frame False {
      }
      frame True {
      }
    }
    n216 = case shown="True" w425 {
      tunnel: w426 -> [_ w533]
      tunnel: [w532 w533] -> w450
      tunnel: w449 -> [w532 _]
      frame False {
      }
      frame True {
      }
    }
    n217 = Wait Until Next ms Multiple(millisecond multiple=u32 100) -> ()  [unwired: 1 out]
    n218 = call <vilib>:"Delimited String to 1D String Array.vi"("delimiter"=",", "delimited string"=w454) -> ("string array"=w530:string[])  [unwired: 9 in]
    n219 = call <vilib>:"Delimited String to 1D String Array.vi"("delimiter"=",", "delimited string"=w450) -> ("string array"=w495:string[])  [unwired: 9 in]
    n220 = call <vilib>:"Delimited String to 1D String Array.vi"("delimiter"=",", "delimited string"=w452) -> ("string array"=w512:string[])  [unwired: 9 in]
    n221 = Index Array(array=w530, index=0) -> ()  [unwired: 1 out]
    n222 = Index Array(array=w530, index=8) -> ()  [unwired: 1 out]
    n223 = Index Array(array=w512, index=0) -> ()  [unwired: 1 out]
    n224 = Index Array(array=w495, index=0) -> ()  [unwired: 1 out]
    n225 = Index Array(array=w512, index=8) -> ()  [unwired: 1 out]
    n226 = Index Array(array=w495, index=8) -> ()  [unwired: 1 out]
    n227 = Index Array(array=w530, index=1) -> (element=w476:string)
    n228 = Index Array(array=w530, index=9) -> ()  [unwired: 1 out]
    n229 = Index Array(array=w512, index=1) -> ()  [unwired: 1 out]
    n230 = Index Array(array=w512, index=9) -> ()  [unwired: 1 out]
    n231 = Index Array(array=w495, index=1) -> (element=w421:string)
    n232 = Index Array(array=w495, index=9) -> ()  [unwired: 1 out]
    n233 = Index Array(array=w530, index=2) -> (element=w473:string)
    n234 = Index Array(array=w530, index=10) -> ()  [unwired: 1 out]
    n235 = Index Array(array=w512, index=2) -> ()  [unwired: 1 out]
    n236 = Index Array(array=w512, index=10) -> ()  [unwired: 1 out]
    n237 = Index Array(array=w495, index=2) -> ()  [unwired: 1 out]
    n238 = Index Array(array=w495, index=10) -> ()  [unwired: 1 out]
    n239 = Fract/Exp String To Number(string=w421) -> (number=→"True_Heading":dbl)  [unwired: 3 in, 1 out]
    n240 = Index Array(array=w530, index=3) -> ()  [unwired: 1 out]
    n241 = Index Array(array=w530, index=11) -> ()  [unwired: 1 out]
    n242 = Index Array(array=w512, index=3) -> ()  [unwired: 1 out]
    n243 = Index Array(array=w495, index=3) -> ()  [unwired: 1 out]
    n244 = Index Array(array=w512, index=11) -> ()  [unwired: 1 out]
    n245 = Index Array(array=w530, index=4) -> (element=w472:string)
    n246 = Index Array(array=w530, index=12) -> ()  [unwired: 1 out]
    n247 = Index Array(array=w512, index=4) -> ()  [unwired: 1 out]
    n248 = Index Array(array=w495, index=4) -> ()  [unwired: 1 out]
    n249 = Index Array(array=w512, index=12) -> ()  [unwired: 1 out]
    n250 = Index Array(array=w530, index=5) -> ()  [unwired: 1 out]
    n251 = Index Array(array=w530, index=13) -> ()  [unwired: 1 out]
    n252 = Index Array(array=w512, index=5) -> ()  [unwired: 1 out]
    n253 = Index Array(array=w495, index=5) -> ()  [unwired: 1 out]
    n254 = Index Array(array=w512, index=13) -> ()  [unwired: 1 out]
    n255 = Index Array(array=w530, index=6) -> (element=→"Fix Position":string)
    n256 = Index Array(array=w530, index=14) -> ()  [unwired: 1 out]
    n257 = Index Array(array=w512, index=6) -> ()  [unwired: 1 out]
    n258 = Index Array(array=w495, index=6) -> ()  [unwired: 1 out]
    n259 = Index Array(array=w512, index=14) -> ()  [unwired: 1 out]
    n260 = Index Array(array=w530, index=7) -> (element=→"Satellited Used":string)
    n261 = Index Array(array=w530, index=15) -> ()  [unwired: 1 out]
    n262 = Index Array(array=w512, index=7) -> (element=w437:string)
    n263 = Scan Value(string=w437, format string="%.3f") -> (value=→"velocity":dbl)  [unwired: 1 in, 1 out]
    n264 = Index Array(array=w495, index=7) -> ()  [unwired: 1 out]
    n265 = Scan Value(string=w476, format string="%.2f") -> (value=→"UTC":dbl)  [unwired: 1 in, 1 out]
    n266 = Scan Value(string=w473, format string="%.2f") -> (value=w459:dbl)  [unwired: 1 in, 1 out]
    "Latitude" <- w459
    n267 = Scan Value(string=w472, format string="%.2f") -> (value=w458:dbl)  [unwired: 1 in, 1 out]
    "Longtitude" <- w458
    n268 = call "dobuncho.vi"("Numeric in"=w459) -> ("Numeric out"=w460:dbl, "String"=→"도분초(lat)":string, "String 2"=→"도(lat)":string)  [unwired: 8 in]
    n269 = call "dobuncho.vi"("Numeric in"=w458) -> ("Numeric out"=w455:dbl, "String"=→"도분초(lon)":string, "String 2"=→"도(lon)":string)  [unwired: 8 in]
    n270 = call "tm_trans.vi"("Long"=w455, "Lat"=w460) -> ("Numeric"=w422:dbl, "out_pt"=w423:dbl)  [unwired: 8 in]
    "TM_Y" <- w422
    "TM_X" <- w423
    n271 = Insert Into Array(array=w446, new element=w422) -> (w445:dbl[])  [unwired: 1 in]
    n272 = Insert Into Array(array=dbl[] [], new element=w423) -> (w442:dbl[])  [unwired: 1 in]
    n273 = Insert Into Array(array=dbl[] [], new element=w422) -> (w441:dbl[])  [unwired: 1 in]
    n274 = Insert Into Array(array=w448, new element=w423) -> (w447:dbl[])  [unwired: 1 in]
    n275 = Bundle("array"=w442, "array"=w441) -> (w440:cluster{"array":dbl[], "array":dbl[]})  [unwired: 1 in]
    n276 = Bundle(w447, w445) -> (w439:cluster{dbl[], dbl[]})  [unwired: 1 in]
    n277 = Build Array(w439, w440) -> (→"XYGraph":cluster{"array":dbl[], "array":dbl[]}[])
  }
  n278 = VISA Flush I/O Buffer(VISA resource name=w2, error in (no error)=w1) -> (VISA resource name out=w5:refnum<visa-resource-name>, error out=w4:errorcluster)  [unwired: 1 in]
  n279 = VISA Close(VISA resource name=w5, error in (no error)=w4) -> (error out=w3:errorcluster)
  n280 = call <vilib>:"Clear Errors.vi"("error in (no error)"=w3) -> ()  [unwired: 5 in, 2 out]
